vi "Trust Actual Server Identity.vi"(8 "error in (no error)":errorcluster, 10 "fingerprint":string, 11 "SSH Client in":refnum<class "PuTTY Client.lvclass">) -> (0 "error out":errorcluster, 2 "permanent?":bool, 3 "SSH Client out":refnum<class "PuTTY Client.lvclass">)   [LabVIEW 2020, in "NI_SSH.lvlib" / "PuTTY Client.lvclass"]
uses:
  <vilib>/net/SSH/Client/PuTTY/PuTTY Client.lvclass
  <vilib>/net/SSH/Client/PuTTY/PuTTY Client.lvclass/PuTTY Client.ctl
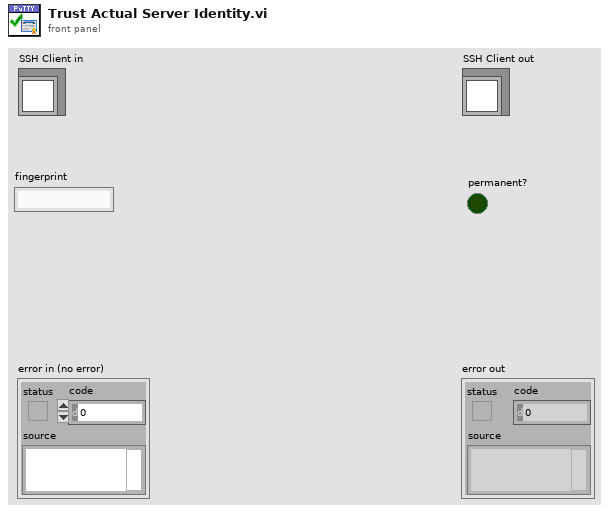
[diagram p1: front panel]
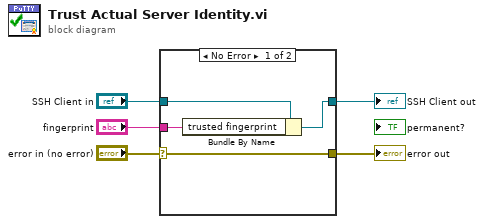
[diagram p0: block diagram]
diagram:
  n1 = case shown="No Error" "error in (no error)" {
    selector: "error in (no error)" -> [w6 w10]
    tunnel: "SSH Client in" -> [w9 w11]
    tunnel: [w7 w11] -> w3
    tunnel: [w6 w10] -> w2
    tunnel: "fingerprint" -> [w8 _]
    frame No Error {
      n2 = Bundle By Name(cluster=w9, "trusted fingerprint"=w8) -> (w7:refnum<class "PuTTY Client.lvclass">)
    }
    frame Error {
    }
  }
  "error out" <- w2
  "SSH Client out" <- w3
